vi "WaypointAndObstaclesPaint.vi"() -> (0 "Obs longs":dbl[](array[numeric]) format="%#_8g", 3 "Obs Lats":dbl[](array[numeric]) format="%#_8g")   [LabVIEW 2014]
panel:
  out "80 by 80 array":u8[][](array[numeric])
  out "Image RGB values":u8[](array[numeric])
  # "Waypoint and Obstacles Paint"
  # "Obstacle latitudes:"
  # "Obstacle Longitudes:"
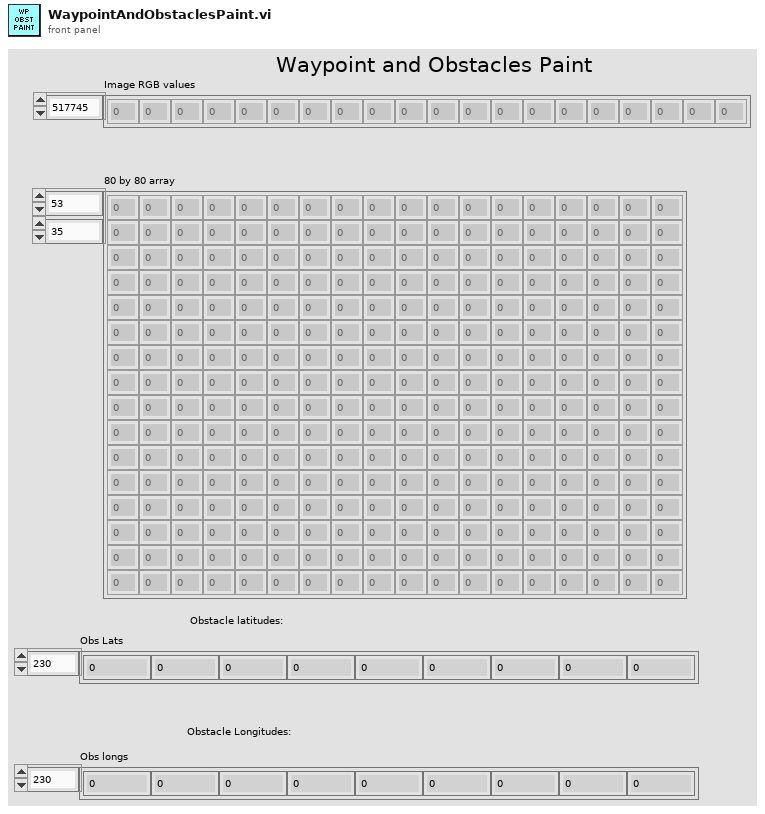
[diagram p1: front panel]
types:
  T1 = typedef "imagedata.ctl" = cluster{"image type":i32, "image depth":i32, "image":u8[], "mask":u8[], "colors":u32[], "Rectangle":cluster{"left":i16, "top":i16, "right":i16, "bottom":i16}}
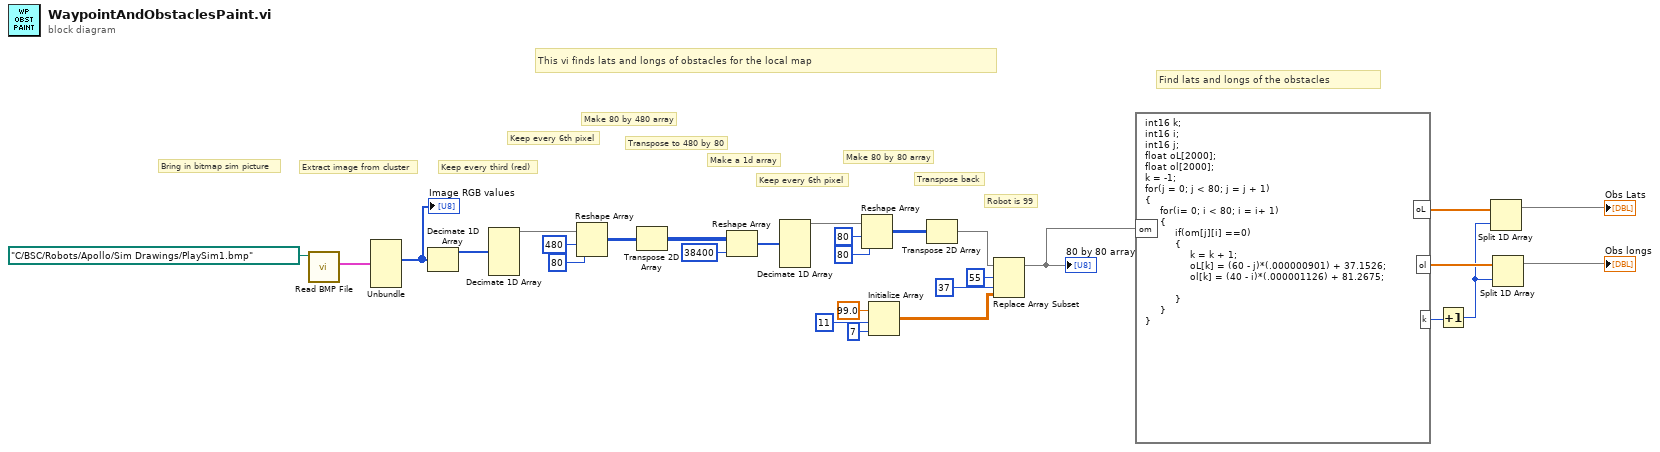
[diagram p0: block diagram]
diagram:
  # "This vi finds lats and longs of obstacles for the local map"
  # "Find lats and longs of the obstacles"
  # "Robot is 99"
  # "Transpose back"
  # "Make 80 by 80 array"
  # "Keep every 6th pixel"
  # "Make a 1d array"
  # "Transpose to 480 by 80"
  # "Make 80 by 480 array"
  # "Keep every 6th pixel"
  # "Keep every third (red)"
  # "Extract image from cluster"
  # "Bring in bitmap sim picture"
  n1 = call <vilib>:"Read BMP File.vi"("path to BMP file"=path "C:/BSC/Robots/Apollo/Sim Drawings/PlaySim1.bmp") -> ("image data"=w28:T1)  [unwired: 8 in, 2 out]
  n2 = Unbundle(w28) -> ("image"=w9:u8[])  [unwired: 5 out]
  "Image RGB values" <- w9
  n3 = Decimate 1D Array(w9) -> (w8:u8[])  [unwired: 2 out]
  n4 = Decimate 1D Array(w8) -> (w27:u8[])  [unwired: 5 out]
  n5 = Reshape Array(w27, 480 ("dimension size"), 80 ("dimension size")) -> (w24:u8[][])
  n6 = Transpose 2D Array(2D array=w24) -> (transposed array=w23:u8[][])
  n7 = Reshape Array(w23, 38400 ("dimension size")) -> (w21:u8[])
  n8 = Decimate 1D Array(w21) -> (w20:u8[])  [unwired: 5 out]
  n9 = Reshape Array(w20, 80 ("dimension size"), 80 ("dimension size")) -> (w17:u8[][])
  n10 = Initialize Array(99.0 ("element"), 11 ("dimension size"), 7 ("dimension size")) -> (w10:dbl[][])
  n11 = Transpose 2D Array(2D array=w17) -> (transposed array=w16:u8[][])
  n12 = Replace Array Subset(array=w16, new element=w10, index (row)=55, index (col)=37 ("disabled index (col)")) -> (w7:u8[][])
  "80 by 80 array" <- w7
  n13 = formula code="int16 k;\nint16 i;\nint16 j;\nfloat oL[2000];\nfloat ol[2000];\nk = -1;\nfor(j = 0; j < 80; j = j + 1)\n{\n     for(i= 0; i < 80; i = i+ 1)\n     {\n          if(om[j][i] ==0)\n          {\n               k = k + 1;\n               oL[k] = (60 - j)*(.000000901) + 37.1526;\n               ol[k] = (40 - i)*(.000001126) + 81.2675;\n          \n          }\n     }\n}"("om"=w7) -> ("oL"=w6:dbl[], "ol"=w4:dbl[], "k"=w2:i16)
  n14 = Increment(x=w2) -> (x+1=w1:i16)
  n15 = Split 1D Array(array=w6, index=w1) -> (first subarray=→"Obs Lats":dbl[])  [unwired: 1 out]
  n16 = Split 1D Array(array=w4, index=w1) -> (first subarray=→"Obs longs":dbl[])  [unwired: 1 out]
